vi "Get Port Speed.vi"(8 "error in":errorcluster, 11 "port ref in":T2 format="%.0x") -> (0 "error out":errorcluster, 2 "speed":T1, 3 "port ref out":T2 format="%.0x")   [LabVIEW 2020, in "AIM ARINC 429 Scripting.lvlib"]
uses:
  <vilib>/NI VeriStand/Custom Device API/Custom Device Item Ref.ctl
  AIM ARINC 429 Scripting.lvlib
  <vilib>/NI VeriStand/Custom Device API/Custom Device API.lvlib
  <vilib>/NI VeriStand/Custom Device API/Get Item Property (U16).vi
  ARINC 429/Constants.vi
  ARINC 429/ARINC 429 Scripting.lvlib
  Shared/Transfer Speed.ctl
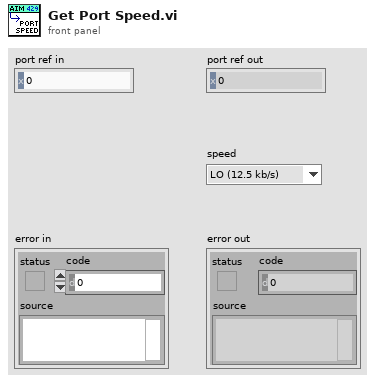
[diagram p1: front panel]
types:
  T1 = typedef "Transfer Speed.ctl" = enum16{"LO (12.5 kb/s)", "HI (100 kb/s)"}
  T2 = typedef "Custom Device API.lvlib/Custom Device Item Ref.ctl" = u64
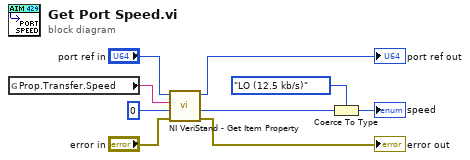
[diagram p0: block diagram]
diagram:
  n1 = global read "Constants.vi" "Prop.Transfer.Speed"() -> (w9:string)
  n2 = call-poly <vilib>:"NI VeriStand - Get Item Property.vi"("error in (no error)"="error in", "Default Value"=u16 0, "Property Name"=w9, "Item Ref in"="port ref in") -> ("error out"=→"error out":errorcluster, "Value"=w4:u16, "Item Ref out"=→"port ref out":T2)  [unwired: 4 in, 1 out]
  n3 = Coerce To Type(0:w4, 1:Transfer_Speed."LO (12.5 kb/s)" ("speed")) -> (2:→"speed":T1)
